vi "XP2i.vi"(4 "error in":T13, 7 "Command":T14) -> (0 "error out":T13, 3 "Response":T11)   [LabVIEW 2018]
uses:
  MOKO_LabViewLibrary/MokoLowLevel/MokoLowLovelControl/MLLC_Command.ctl
  MOKO_LabViewLibrary/MokoLowLevel/MokoLowLovelControl/MLLC_Error.ctl
  MOKO_LabViewLibrary/MokoLowLevel/MokoLowLovelControl/MLLC_Mode.ctl
  MOKO_LabViewLibrary/MokoLowLevel/MokoLowLovelControl/MLLC_Response.ctl
  MOKO_LabViewLibrary/MokoLowLevel/MokoLowLovelControl/MLLC_DriverName.ctl
  MOKO_LabViewLibrary/MokoLowLevel/MokoLowLovelControl/MLLC_ResponseInit.ctl
  MOKO_LabViewLibrary/MokoLowLevel/MokoLowLovelControl/MLLC_Request.ctl
  MOKO_LabViewLibrary/MokoLowLevel/MokoLowLovelControl/MLLC_ErrorCode.ctl
  MOKO_LabViewLibrary/MokoLowLevel/MokoLowLovelControl/MLLC_ConnectCluster.ctl
  MOKO_LabViewLibrary/MokoLowLevel/MokoLowLovelControl/MLLC_InterfaceType.ctl
  MOKO_LabViewLibrary/MokoLowLevel/MokoLowLovelControl/MLLC_OpenedSession.ctl
  MOKO_LabViewLibrary/MokoLowLevel/MokoLowLovelControl/MLLC_InterfaceSettings.ctl
  MOKO_LabViewLibrary/MokoLowLevel/MokoLowLovelControl/MLLC_InterfaceKind.ctl
  MOKO_LabViewLibrary/MokoLowLevel/MokoLowLovelControl/MLLC_Rs232Settings.ctl
panel:
  in  "Settings":T6={"Saved Data"=variant, "Permanent data"={"Connect"={"InterfaceType"=enum."VISA", "OpenedSession"="COM4", "InterfaceSettings"={"Interface"=enum."RS232", "EOS 4 read"=enum."Default (=EOS 4 write)", "EOS 4 write"=enum."CR (\\r)", "TMO, ms"=2000, "Sett"=variant(cluster{"Baud Rate":u32, "Data Bits":u16, "Parity":u16, "Stop Bits":u16, "Flow Control":u16, "Eho":bool} {"Baud Rate"=75, "Data Bits"=0, "Parity"=0, "Stop Bits"=0, "Flow Control"=0, "Eho"=FALSE})}}}}
  in  "Error Code":T7=5420
  in  "Request":T8="?MOD"
  in  "ResponseInit":T9="XP2I"
  in  "Driver Name":T10="Crystal XP2"
  in  "Mode":T12=enum."Check"
  # "XP2i"
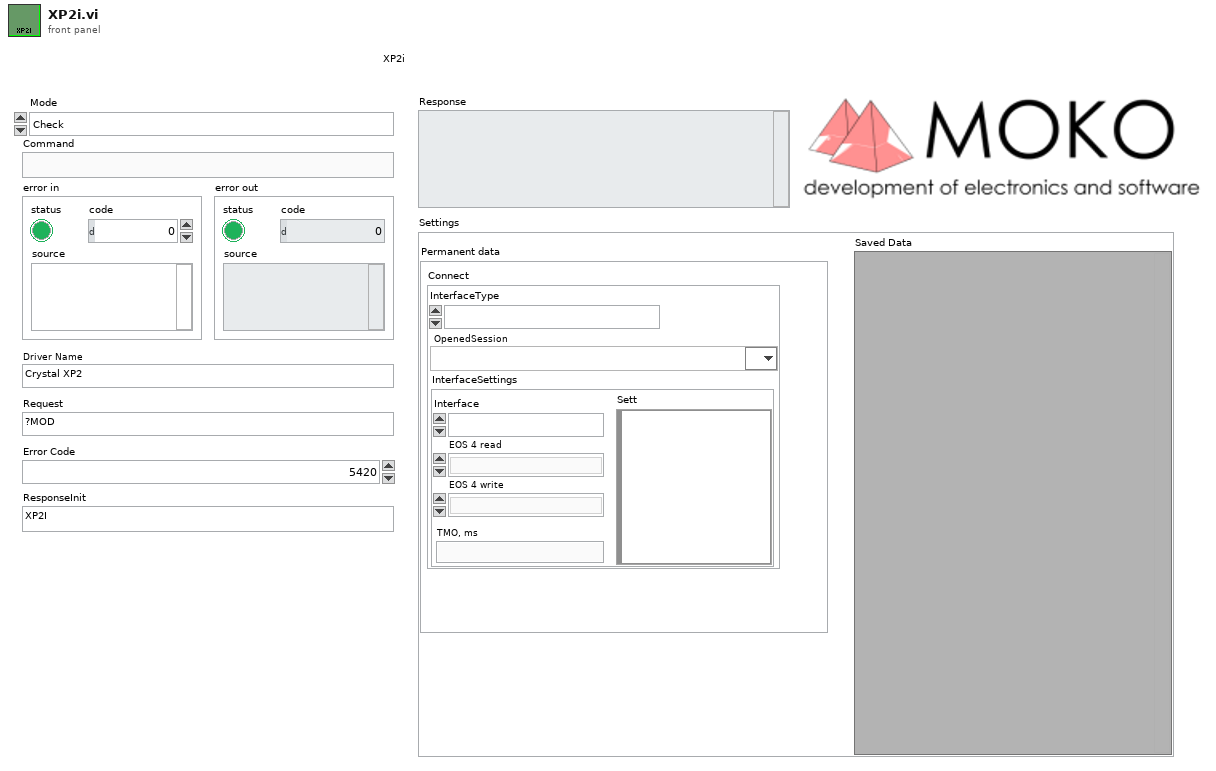
[diagram p1: front panel]
types:
  T1 = typedef "MLLC_ConnectCluster.ctl" = cluster{"InterfaceType":T2, "OpenedSession":T3, "InterfaceSettings":T4}
  T2 = typedef "MLLC_InterfaceType.ctl" = enum16{"VISA", "Prologix USB-GPIB"}
  T3 = typedef "MLLC_OpenedSession.ctl" = refnum<visa-resource-name>
  T4 = typedef "MLLC_InterfaceSettings.ctl" = cluster{"Interface":T5, "EOS 4 read":enum16{"Default (=EOS 4 write)", "CR (\\r)", "LF (\\n)", "None"}, "EOS 4 write":enum16{"CR+LF (\\r\\n)", "CR (\\r)", "LF (\\n)", "None"}, "TMO, ms":i32, "Sett":variant}
  T5 = typedef "MLLC_InterfaceKind.ctl" = enum16{"RS232", "GPIB", "USB", "Ethernet", "another"}
  T6 = cluster{"Saved Data":variant, "Permanent data":cluster{"Connect":T1}}
  T7 = typedef "MLLC_ErrorCode.ctl" = u32
  T8 = typedef "MLLC_Request.ctl" = string
  T9 = typedef "MLLC_ResponseInit.ctl" = string
  T10 = typedef "MLLC_DriverName.ctl" = string
  T11 = typedef "MLLC_Response.ctl" = string
  T12 = typedef "MLLC_Mode.ctl" = enum16{"get", "set", "close", "Init", "Check"}
  T13 = typedef "MLLC_Error.ctl" = errorcluster
  T14 = typedef "MLLC_Command.ctl" = string
  T15 = typedef "MLLC_Rs232Settings.ctl" = cluster{"Baud Rate":u32, "Data Bits":u16, "Parity":u16, "Stop Bits":u16, "Flow Control":u16, "Eho":bool}
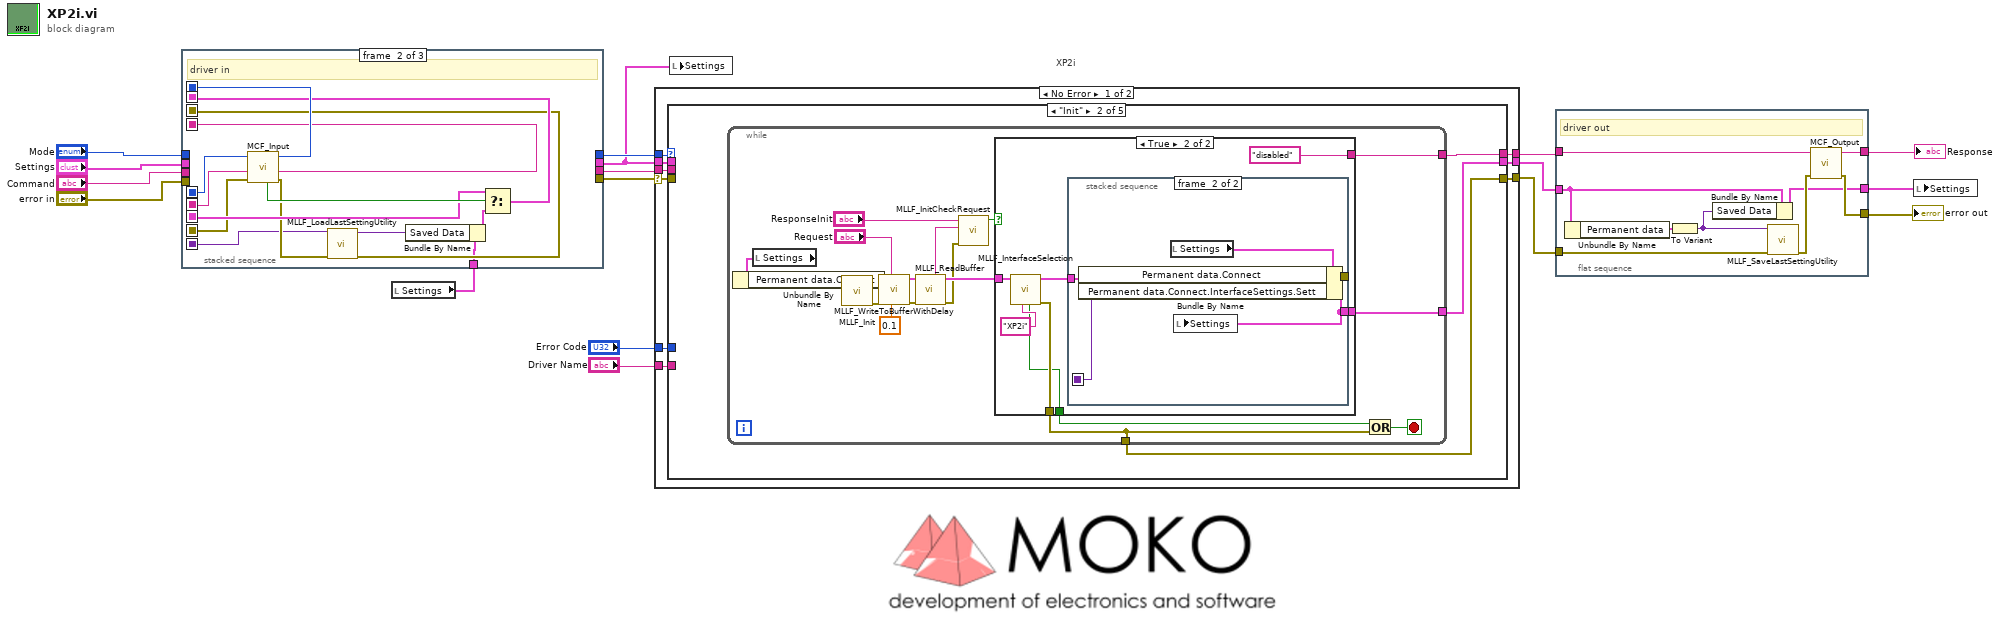
[diagram p0: block diagram]
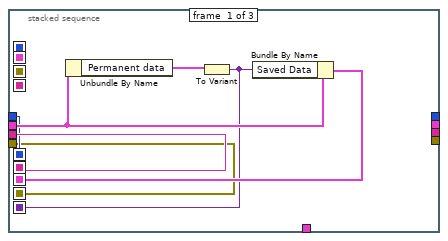
[diagram p2: hidden frame]
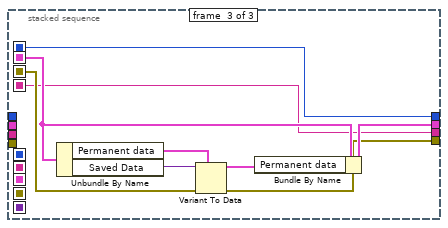
[diagram p3: hidden frame]
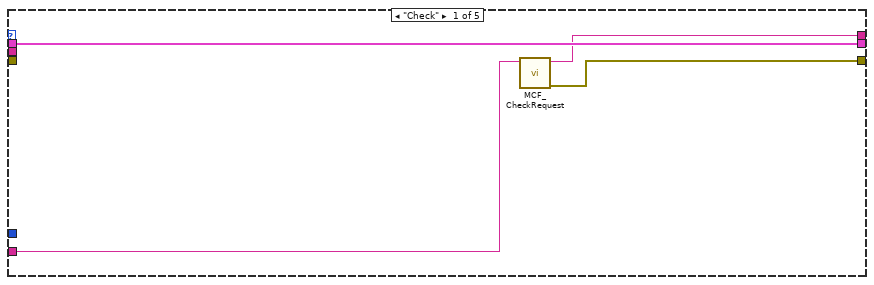
[diagram p4: hidden frame]
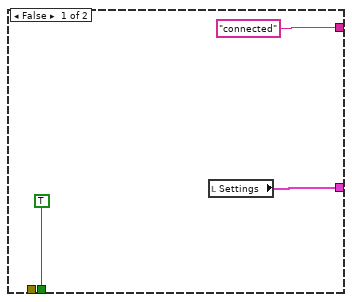
[diagram p5: hidden frame]
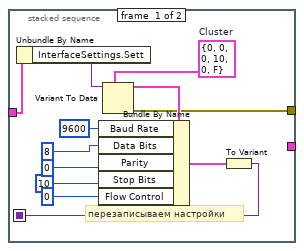
[diagram p6: hidden frame]
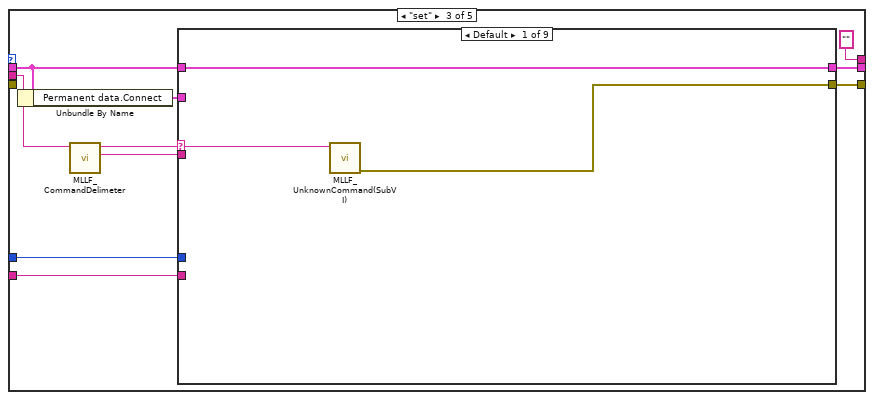
[diagram p7: hidden frame]
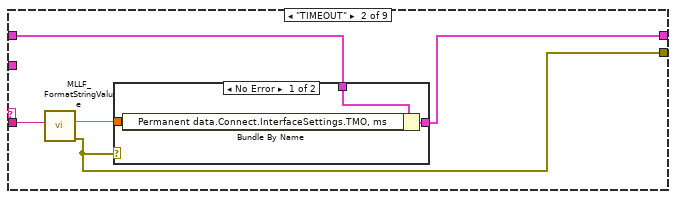
[diagram p8: hidden frame]
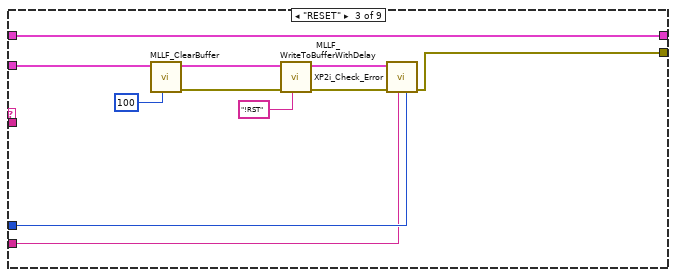
[diagram p10: hidden frame]
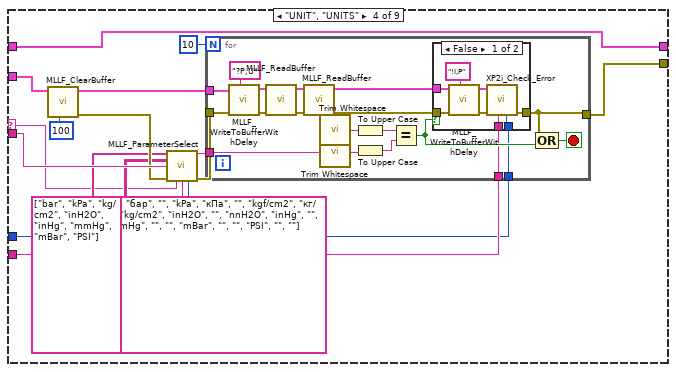
[diagram p11: hidden frame]
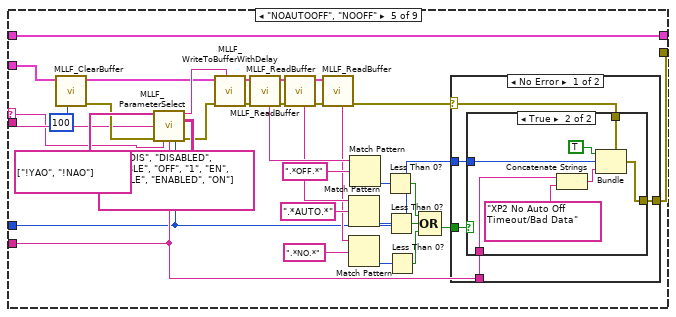
[diagram p13: hidden frame]
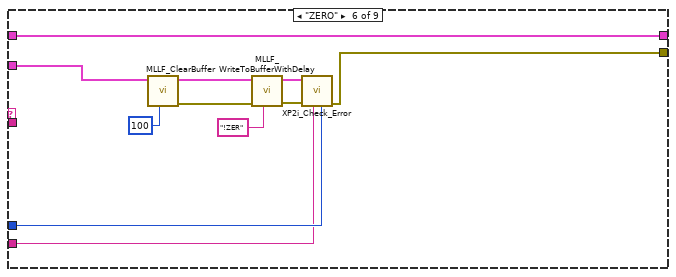
[diagram p16: hidden frame]
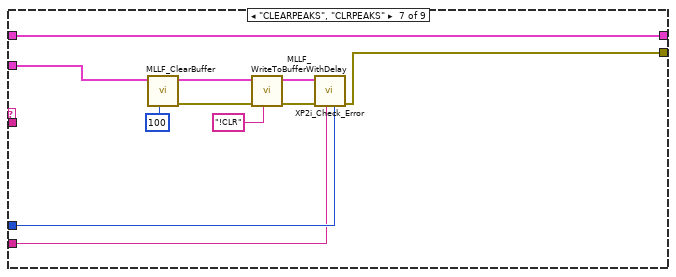
[diagram p17: hidden frame]
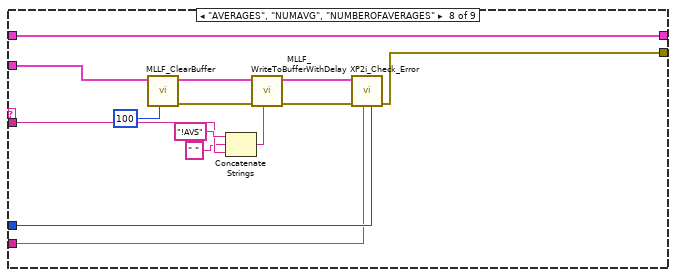
[diagram p18: hidden frame]
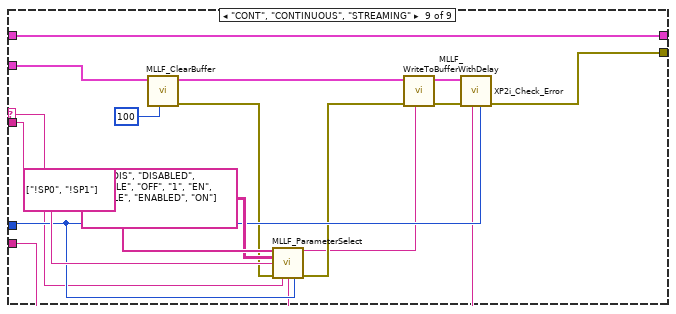
[diagram p19: hidden frame]
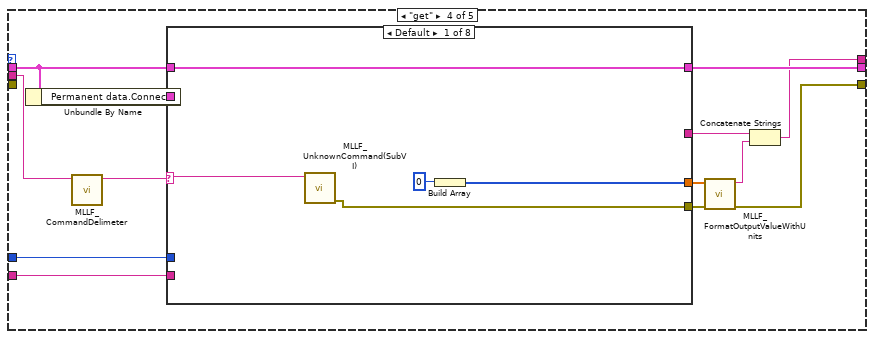
[diagram p20: hidden frame]
diagram:
  # "XP2i"
  n1 = local read "Settings"() -> (w7:T6)
  n2 = stacked-sequence {
    seq-local: [w20 _ _] -> [_ w36 _]
    seq-local: [w19 _ _] -> [_ w37 _]
    seq-local: [w22 _ _] -> [_ w32 _]
    seq-local: [w18 _ _] -> [_ w31 _]
    seq-local: [w21 _ _] -> [_ w27 _]
    seq-local: [_ w28 _] -> [_ _ w44]
    seq-local: [_ w38 _] -> [_ _ w41]
    seq-local: [_ w35 _] -> [_ _ w40]
    seq-local: [_ w34 _] -> [_ _ w45]
    tunnel: "Command" -> [w20 _ _]
    tunnel: "Mode" -> [w19 _ _]
    tunnel: "error in" -> [w18 _ _]
    tunnel: "Settings" -> [w23 _ _]
    tunnel: w7 -> [_ w26 _]
    tunnel: [_ _ w40] -> w9
    tunnel: [_ _ w43] -> w10
    tunnel: [_ _ w42] -> w8
    tunnel: [_ _ w41] -> w11
    frame #0 {
      n3 = Unbundle By Name(w23) -> ("Permanent data"=w24:cluster{"Connect":T1})
      n4 = To Variant(anything=w24) -> (Variant=w21:variant)
      n5 = Bundle By Name(cluster=w23, "Saved Data"=w21) -> (w22:T6)
    }
    frame #1 {
      # "driver in"
      n6 = call "MCF_Input.vi"("Error In"=w31, "Command in"=w36, "Mode in"=w37) -> ("Error Out"=w30:errorcluster, "Command out"=w35:string, "Mode out"=w38:T12, "Boolean"=w33:bool)  [unwired: 5 in]
      n7 = call "MLLF_LoadLastSettingUtility.vi"("Error In"=w30, "Save data in"=w27) -> ("Error Out"=w28:errorcluster, "Save data out"=w25:variant)  [unwired: 8 in]
      n8 = Bundle By Name(cluster=w26, "Saved Data"=w25) -> (w29:T6)
      n9 = Select(t=w32, s=w33, f=w29) -> (s? t:f=w34:T6)
    }
    frame #2 {
      n10 = Unbundle By Name(w45) -> ("Permanent data"=w46:cluster{"Connect":T1}, "Saved Data"=w39:variant)
      n11 = Variant To Data(error in=w44, type=w46, Variant=w39) -> (data=w47:cluster{"Connect":T1}, error out=w42:errorcluster)
      n12 = Bundle By Name(cluster=w45, "Permanent data"=w47) -> (w43:T6)
    }
  }
  n13 = case shown="No Error" w8 {
    selector: w8 -> [w53 w409]
    tunnel: [w48 w409] -> w4
    tunnel: w11 -> [w56 _]
    tunnel: [w55 _] -> w6
    tunnel: w9 -> [w54 _]
    tunnel: w10 -> [w50 w408]
    tunnel: "Error Code" -> [w52 _]
    tunnel: "Driver Name" -> [w51 _]
    tunnel: [w49 w408] -> w5
    frame No Error {
      n14 = case shown="\"Init\"" w56 {
        tunnel: [w58 w63 "" ("Output String") w293 "" ("Output String")] -> w55
        tunnel: w54 -> [_ _ w110 w286 _]
        tunnel: w53 -> [_ _ _ _ _]
        tunnel: w52 -> [_ _ w117 w296 _]
        tunnel: w51 -> [w59 _ w114 w295 _]
        tunnel: w50 -> [w60 _ w116 w297 w406]
        tunnel: [w60 w62 w115 w294 w406] -> w49
        tunnel: [w57 w61 w113 w287 w405] -> w48
        frame "Check" {
          n15 = call "MCF_CheckRequest.vi"("Driver Name"=w59) -> ("Error Out"=w57:errorcluster, "Output String"=w58:string)  [unwired: 9 in]
        }
        frame "Init" {
          n16 = while {
            tunnel: [w76] -> w61
            tunnel: [w73] -> w63
            tunnel: [w72] -> w62
            stop <- w78 stop-if-true
            n17 = local read "Settings"() -> (w66:T6)
            n18 = Unbundle By Name(w66) -> ("Permanent data.Connect"=w65:T1)
            n19 = call "MLLF_Init.vi"("DriverConnect in"=w65) -> ("Error Out"=w80:errorcluster, "DriverConnect out"=w79:T1)  [unwired: 7 in]
            n20 = call "MLLF_WriteToBufferWithDelay.vi"("Delay Time ( 0,05 s)"=0.1 ("Delay Time (s)"), "Command"="Request", "Error In"=w80, "DriverConnect in"=w79) -> ("Error Out"=w75:errorcluster, "DriverConnect out"=w64:T1)  [unwired: 6 in]
            n21 = call "MLLF_ReadBuffer.vi"("Error In"=w75, "DriverConnect in"=w64) -> ("Error Out"=w70:errorcluster, "DriverConnect out"=w81:T1, "String"=w71:string)  [unwired: 6 in]
            n22 = call "MLLF_InitCheckRequest.vi"("error in (no error)"=w70, "Answer"=w71, "Response Init"="ResponseInit") -> ("Design"=w69:bool)  [unwired: 5 in, 3 out]
            n23 = case shown="True" w69 {
              tunnel: w81 -> [_ w90]
              tunnel: [TRUE w86] -> w77
              tunnel: [_ w91] -> w76
              tunnel: ["connected" "disabled"] -> w73
              tunnel: [w82 w85] -> w72
              frame False {
                n24 = local read "Settings"() -> (w82:T6)
              }
              frame True {
                n25 = call "MLLF_InterfaceSelection.vi"("Driver Name"="XP2i" ("String"), "DriverConnect in"=w90) -> ("error out"=w91:T13, "DriverConnect out"=w89:T1, "stop init?"=w86:bool)  [unwired: 7 in]
                n26 = stacked-sequence {
                  seq-local: [w95 _] -> [_ w104]
                  tunnel: w89 -> [w93 w105]
                  tunnel: [w96 _] -> _
                  tunnel: [_ w106] -> w85
                  frame #0 {
                    w97 = T15 {"Baud Rate"=0, "Data Bits"=0, "Parity"=0, "Stop Bits"=10, "Flow Control"=0, "Eho"=FALSE}  # Cluster
                    # "перезаписываем настройки"
                    n27 = Unbundle By Name(w93) -> ("InterfaceSettings.Sett"=w92:variant)
                    n28 = Variant To Data(type=w97, Variant=w92) -> (data=w98:T15, error out=w96:errorcluster)  [unwired: 1 in]
                    n29 = Bundle By Name(cluster=w98, "Baud Rate"=u32 9600, "Data Bits"=u16 8 ("Serial Settings:Data Bits"), "Parity"=u16 0 ("Serial Settings:Parity"), "Stop Bits"=u16 10 ("Serial Settings:Stop Bits"), "Flow Control"=u16 0 ("Serial Settings:Flow Control")) -> (w103:T15)
                    n30 = To Variant(anything=w103) -> (Variant=w95:variant)
                  }
                  frame #1 {
                    n31 = local read "Settings"() -> (w107:T6)
                    n32 = Bundle By Name(cluster=w107, "Permanent data.Connect"=w105, "Permanent data.Connect.InterfaceSettings.Sett"=w104) -> (w106:T6)
                    n33 = local write "Settings"(w106) -> ()
                  }
                }
              }
            }
            n34 = Or(x=w77, y=w76) -> (x .or. y?=w78:bool)
          }
        }
        frame "set" {
          n35 = Unbundle By Name(w116) -> ("Permanent data.Connect"=w111:T1)
          n36 = call "MLLF_CommandDelimeter.vi"("command with param"=w110) -> ("param 1"=w108:string, "command"=w109:string)  [unwired: 6 in, 3 out]
          n37 = case shown="Default" w109 {
            selector: w109 -> [w119 _ _ w141 w185 _ _ _ w270]
            tunnel: w108 -> [_ w123 _ w153 w193 _ _ w260 w279]
            tunnel: w117 -> [_ _ w138 w151 w195 w238 w249 w264 w278]
            tunnel: w116 -> [w120 w124 w140 w144 w218 w243 w254 w268 w284]
            tunnel: [w120 w125 w140 w144 w218 w243 w254 w268 w284] -> w115
            tunnel: w114 -> [_ _ w137 w152 w196 w237 w248 w263 w269]
            tunnel: w111 -> [_ _ w131 w143 w187 w234 w245 w256 w272]
            tunnel: [w118 w121 w130 w142 w186 w233 w244 w255 w271] -> w113
            frame Default {
              n38 = call "MLLF_UnknownCommand(SubVI).vi"("Unknown command"=w119) -> ("error out"=w118:errorcluster)  [unwired: 10 in]
            }
            frame "TIMEOUT" {
              n39 = call "MLLF_FormatStringValue.vi"("String Value"=w123) -> ("error out"=w121:T13, "number"=w122:dbl)  [unwired: 8 in, 1 out]
              n40 = case shown="No Error" w121 {
                tunnel: [w128 w129] -> w125
                tunnel: w124 -> [w127 w129]
                tunnel: w122 -> [w126 _]
                frame No Error {
                  n41 = Bundle By Name(cluster=w127, "Permanent data.Connect.InterfaceSettings.TMO, ms"=w126) -> (w128:T6)
                }
                frame Error {
                }
              }
            }
            frame "RESET" {
              n42 = call "MLLF_ClearBuffer.vi"("Timeout"=u32 100, "DriverConnect in"=w131) -> ("Error Out"=w135:errorcluster, "DriverConnect out"=w134:T1)  [unwired: 6 in, 1 out]
              n43 = call "MLLF_WriteToBufferWithDelay.vi"("Command"="!RST" ("String"), "Error In"=w135, "DriverConnect in"=w134) -> ("Error Out"=w133:errorcluster, "DriverConnect out"=w139:T1)  [unwired: 7 in]
              n44 = call "XP2i_Check_Error.vi"("Error Code"=w138, "Driver Name"=w137, "Error In"=w133, "DriverConnect in"=w139) -> ("Error Out"=w130:errorcluster)  [unwired: 6 in, 1 out]
            }
            frame "UNIT", "UNITS" {
              n45 = call "MLLF_ClearBuffer.vi"("Timeout"=u32 100, "DriverConnect in"=w143) -> ("Error Out"=w150:errorcluster, "DriverConnect out"=w154:T1)  [unwired: 6 in, 1 out]
              n46 = call "MLLF_ParameterSelect.vi"("Command to equipment"=string[] ["bar", "kPa", "kg/cm2", "inH2O", "inHg", "mmHg", "mBar", "PSI"] ("Parameters 2 equipment"), "Names"=string[][] [["bar", "бар", ""], ["kPa", "кПа", ""], ["kgf/cm2", "кг/см2", "kg/cm2"], ["inH2O", "", "nnH2O"], ["inHg", "", ""], ["mmHg", "", ""], ["mBar", "", ""], ["PSI", "", ""]], "Input"=w153, "Error In"=w150, "Command"=w141, "Driver Name"=w152, "Error Code"=w151) -> ("Choice"=w148:string, "Error Out"=w149:errorcluster)  [unwired: 7 in]
              n47 = for {
                N: 10 -> [_]
                tunnel: w154 -> [w165]
                tunnel: [w159] -> w142
                tunnel: w148 -> [w163]
                tunnel: w152 -> [w157]
                tunnel: w151 -> [w156]
                tunnel: w149 -> [w164]
                stop <- w171 stop-if-true
                n48 = call "MLLF_WriteToBufferWithDelay.vi"("Command"="?P,U" ("String"), "Error In"=w164, "DriverConnect in"=w165) -> ("Error Out"=w167:errorcluster, "DriverConnect out"=w174:T1)  [unwired: 7 in]
                n49 = call "MLLF_ReadBuffer.vi"("Error In"=w167, "DriverConnect in"=w174) -> ("Error Out"=w170:errorcluster, "DriverConnect out"=w169:T1)  [unwired: 6 in, 1 out]
                n50 = call "MLLF_ReadBuffer.vi"("Error In"=w170, "DriverConnect in"=w169) -> ("Error Out"=w160:errorcluster, "DriverConnect out"=w161:T1, "String"=w168:string)  [unwired: 6 in]
                n51 = call <vilib>:"Trim Whitespace.vi"("string"=w168) -> ("trimmed string"=w166:string)  [unwired: 1 in]
                n52 = call <vilib>:"Trim Whitespace.vi"("string"=w163) -> ("trimmed string"=w162:string)  [unwired: 1 in]
                n53 = To Upper Case(1:w166) -> (0:w173:string)
                n54 = To Upper Case(1:w162) -> (0:w172:string)
                n55 = Equal?(x=w173, y=w172) -> (x = y?=w158:bool)
                n56 = case shown="False" w158 {
                  tunnel: w161 -> [w180 _]
                  tunnel: w160 -> [w179 w184]
                  tunnel: [w178 w184] -> w159
                  tunnel: w157 -> [w177 _]
                  tunnel: w156 -> [w176 _]
                  frame False {
                    n57 = call "MLLF_WriteToBufferWithDelay.vi"("Command"="!I,P" ("String"), "Error In"=w179, "DriverConnect in"=w180) -> ("Error Out"=w181:errorcluster, "DriverConnect out"=w182:T1)  [unwired: 7 in]
                    n58 = call "XP2i_Check_Error.vi"("Error Code"=w176, "Driver Name"=w177, "Error In"=w181, "DriverConnect in"=w182) -> ("Error Out"=w178:errorcluster)  [unwired: 6 in, 1 out]
                  }
                  frame True {
                  }
                }
                n59 = Compound Arithmetic op=OR(w159, w158) -> (w171:bool)
              }
            }
            frame "NOAUTOOFF", "NOOFF" {
              n60 = call "MLLF_ClearBuffer.vi"("Timeout"=u32 100, "DriverConnect in"=w187) -> ("Error Out"=w194:errorcluster, "DriverConnect out"=w190:T1)  [unwired: 6 in, 1 out]
              n61 = call "MLLF_ParameterSelect.vi"("Command to equipment"=string[] ["!YAO", "!NAO"] ("Names"), "Names"=string[][] [["0", "DIS", "DISABLED", "DISABLE", "OFF"], ["1", "EN", "ENABLE", "ENABLED", "ON"]], "Input"=w193, "Error In"=w194, "Command"=w185, "Driver Name"=w196, "Error Code"=w195) -> ("Choice"=w192:string, "Error Out"=w191:errorcluster)  [unwired: 7 in]
              n62 = call "MLLF_WriteToBufferWithDelay.vi"("Command"=w192, "Error In"=w191, "DriverConnect in"=w190) -> ("Error Out"=w188:errorcluster, "DriverConnect out"=w217:T1)  [unwired: 7 in]
              n63 = call "MLLF_ReadBuffer.vi"("Error In"=w188, "DriverConnect in"=w217) -> ("Error Out"=w216:errorcluster, "DriverConnect out"=w215:T1, "String"=w203:string)  [unwired: 6 in]
              n64 = call "MLLF_ReadBuffer.vi"("Error In"=w216, "DriverConnect in"=w215) -> ("Error Out"=w214:errorcluster, "DriverConnect out"=w213:T1, "String"=w202:string)  [unwired: 6 in]
              n65 = call "MLLF_ReadBuffer.vi"("Error In"=w214, "DriverConnect in"=w213) -> ("Error Out"=w200:errorcluster, "String"=w201:string)  [unwired: 6 in, 1 out]
              n66 = Match Pattern(string=w202, regular expression=".*AUTO.*") -> (offset past match=w208:i32)  [unwired: 1 in, 3 out]
              n67 = Match Pattern(string=w201, regular expression=".*NO.*") -> (offset past match=w209:i32)  [unwired: 1 in, 3 out]
              n68 = Match Pattern(string=w203, regular expression=".*OFF.*") -> (offset past match=w207:i32)  [unwired: 1 in, 3 out]
              n69 = Less Than 0?(x=w207) -> (x < 0?=w210:bool)
              n70 = Less Than 0?(x=w208) -> (x < 0?=w211:bool)
              n71 = Less Than 0?(x=w209) -> (x < 0?=w212:bool)
              n72 = Compound Arithmetic op=OR(w210, w211, w212) -> (w199:bool)
              n73 = case shown="No Error" w200 {
                selector: w200 -> [w219 w232]
                tunnel: [w223 w232] -> w186
                tunnel: w199 -> [w222 _]
                tunnel: w195 -> [w221 _]
                tunnel: w196 -> [w220 _]
                frame No Error {
                  n74 = case shown="True" w222 {
                    tunnel: [w224 w230] -> w223
                    tunnel: w221 -> [_ w229]
                    tunnel: w220 -> [_ w227]
                    tunnel: w219 -> [w224 w225]
                    frame False {
                    }
                    frame True {
                      n75 = Concatenate Strings(w227, "XP2 No Auto Off Timeout/Bad Data") -> (w226:string)
                      n76 = Bundle(cluster=w225, "status"=TRUE, "code"=w229, "source"=w226) -> (w230:errorcluster)
                    }
                  }
                }
                frame Error {
                }
              }
            }
            frame "ZERO" {
              n77 = call "MLLF_ClearBuffer.vi"("Timeout"=u32 100, "DriverConnect in"=w234) -> ("Error Out"=w241:errorcluster, "DriverConnect out"=w240:T1)  [unwired: 6 in, 1 out]
              n78 = call "MLLF_WriteToBufferWithDelay.vi"("Command"="!ZER" ("String"), "Error In"=w241, "DriverConnect in"=w240) -> ("Error Out"=w235:errorcluster, "DriverConnect out"=w239:T1)  [unwired: 7 in]
              n79 = call "XP2i_Check_Error.vi"("Error Code"=w238, "Driver Name"=w237, "Error In"=w235, "DriverConnect in"=w239) -> ("Error Out"=w233:errorcluster)  [unwired: 6 in, 1 out]
            }
            frame "CLEARPEAKS", "CLRPEAKS" {
              n80 = call "MLLF_ClearBuffer.vi"("Timeout"=u32 100, "DriverConnect in"=w245) -> ("Error Out"=w252:errorcluster, "DriverConnect out"=w251:T1)  [unwired: 6 in, 1 out]
              n81 = call "MLLF_WriteToBufferWithDelay.vi"("Command"="!CLR" ("String"), "Error In"=w252, "DriverConnect in"=w251) -> ("Error Out"=w247:errorcluster, "DriverConnect out"=w250:T1)  [unwired: 7 in]
              n82 = call "XP2i_Check_Error.vi"("Error Code"=w249, "Driver Name"=w248, "Error In"=w247, "DriverConnect in"=w250) -> ("Error Out"=w244:errorcluster)  [unwired: 6 in, 1 out]
            }
            frame "AVERAGES", "NUMAVG", "NUMBEROFAVERAGES" {
              n83 = call "MLLF_ClearBuffer.vi"("Timeout"=u32 100, "DriverConnect in"=w256) -> ("Error Out"=w267:errorcluster, "DriverConnect out"=w266:T1)  [unwired: 6 in, 1 out]
              n84 = Concatenate Strings("!AVS" ("String"), " " ("string"), w260) -> (w261:string)
              n85 = call "MLLF_WriteToBufferWithDelay.vi"("Command"=w261, "Error In"=w267, "DriverConnect in"=w266) -> ("Error Out"=w258:errorcluster, "DriverConnect out"=w265:T1)  [unwired: 7 in]
              n86 = call "XP2i_Check_Error.vi"("Error Code"=w264, "Driver Name"=w263, "Error In"=w258, "DriverConnect in"=w265) -> ("Error Out"=w255:errorcluster)  [unwired: 6 in, 1 out]
            }
            frame "CONT", "CONTINUOUS", "STREAMING" {
              n87 = call "MLLF_ClearBuffer.vi"("Timeout"=u32 100, "DriverConnect in"=w272) -> ("Error Out"=w277:errorcluster, "DriverConnect out"=w283:T1)  [unwired: 6 in, 1 out]
              n88 = call "MLLF_ParameterSelect.vi"("Command to equipment"=string[] ["!SP0", "!SP1"] ("Names"), "Names"=string[][] [["0", "DIS", "DISABLED", "DISABLE", "OFF"], ["1", "EN", "ENABLE", "ENABLED", "ON"]], "Input"=w279, "Error In"=w277, "Command"=w270, "Driver Name"=w269, "Error Code"=w278) -> ("Choice"=w275:string, "Error Out"=w276:errorcluster)  [unwired: 7 in]
              n89 = call "MLLF_WriteToBufferWithDelay.vi"("Command"=w275, "Error In"=w276, "DriverConnect in"=w283) -> ("Error Out"=w274:errorcluster, "DriverConnect out"=w282:T1)  [unwired: 7 in]
              n90 = call "XP2i_Check_Error.vi"("Error Code"=w278, "Driver Name"=w269, "Error In"=w274, "DriverConnect in"=w282) -> ("Error Out"=w271:errorcluster)  [unwired: 6 in, 1 out]
            }
          }
        }
        frame "get" {
          n91 = Unbundle By Name(w297) -> ("Permanent data.Connect"=w288:T1)
          n92 = call "MLLF_CommandDelimeter.vi"("command with param"=w286) -> ("command"=w285:string)  [unwired: 6 in, 4 out]
          n93 = case shown="Default" w285 {
            selector: w285 -> [w299 _ _ _ _ _ _ _]
            tunnel: [w298 _ w314 w328 w345 w362 w379 w396] -> w292
            tunnel: w296 -> [_ _ _ _ _ _ _ _]
            tunnel: [w302 w305 w318 w335 w352 w369 w386 w403] -> w294
            tunnel: w297 -> [w302 w305 w318 w335 w352 w369 w386 w403]
            tunnel: [w300 w303 _ w332 w349 w366 w383 w400] -> w291
            tunnel: w295 -> [_ _ _ _ _ _ _ _]
            tunnel: [_ _ w309 _ _ _ _ _] -> w289
            tunnel: w288 -> [_ _ w306 w319 w336 w353 w370 w387]
            frame Default {
              n94 = call "MLLF_UnknownCommand(SubVI).vi"("Unknown command"=w299) -> ("error out"=w298:errorcluster)  [unwired: 10 in]
              n95 = Build Array(0 ("TimeOut")) -> (w300:i32[])
            }
            frame "TIMEOUT" {
              n96 = Unbundle By Name(w305) -> ("Permanent data.Connect.InterfaceSettings.TMO, ms"=w304:i32)
              n97 = Build Array(w304) -> (w303:i32[])
            }
            frame "PRESSURE" {
              n98 = call "MLLF_ClearBuffer.vi"("Timeout"=u32 100, "DriverConnect in"=w306) -> ("Error Out"=w315:errorcluster, "DriverConnect out"=w316:T1)  [unwired: 6 in, 1 out]
              n99 = call "MLLF_WriteToBufferWithDelay.vi"("Command"="?PRE" ("String"), "Error In"=w315, "DriverConnect in"=w316) -> ("Error Out"=w308:errorcluster, "DriverConnect out"=w313:T1)  [unwired: 7 in]
              n100 = call "MLLF_ReadBuffer.vi"("Error In"=w308, "DriverConnect in"=w313) -> ("Error Out"=w314:errorcluster, "String"=w312:string)  [unwired: 6 in, 1 out]
              n101 = Match Pattern(string=w312, regular expression=",") -> (before substring=w310:string)  [unwired: 1 in, 3 out]
              n102 = call <vilib>:"Trim Whitespace.vi"("string"=w310) -> ("trimmed string"=w309:string)  [unwired: 1 in]
            }
            frame "PRESSUREHIGH" {
              n103 = call "MLLF_ClearBuffer.vi"("Timeout"=u32 100, "DriverConnect in"=w319) -> ("Error Out"=w329:errorcluster, "DriverConnect out"=w330:T1)  [unwired: 6 in, 1 out]
              n104 = call "MLLF_WriteToBufferWithDelay.vi"("Command"="?P,H" ("String"), "Error In"=w329, "DriverConnect in"=w330) -> ("Error Out"=w321:errorcluster, "DriverConnect out"=w325:T1)  [unwired: 7 in]
              n105 = call "MLLF_ReadBuffer.vi"("Error In"=w321, "DriverConnect in"=w325) -> ("Error Out"=w324:errorcluster, "DriverConnect out"=w323:T1, "String"=w322:string)  [unwired: 6 in]
              n106 = call "MLLF_ReadBuffer.vi"("Error In"=w324, "DriverConnect in"=w323) -> ("Error Out"=w328:errorcluster)  [unwired: 6 in, 2 out]
              n107 = Match Pattern(string=w322, regular expression=",") -> (before substring=w326:string)  [unwired: 1 in, 3 out]
              n108 = Fract/Exp String To Number(use system decimal point (T)=FALSE, string=w326) -> (number=w333:dbl)  [unwired: 2 in, 1 out]
              n109 = Build Array(w333) -> (w332:dbl[])
            }
            frame "PRESSURELOW" {
              n110 = call "MLLF_ClearBuffer.vi"("Timeout"=u32 100, "DriverConnect in"=w336) -> ("Error Out"=w346:errorcluster, "DriverConnect out"=w347:T1)  [unwired: 6 in, 1 out]
              n111 = call "MLLF_WriteToBufferWithDelay.vi"("Command"="?P,L" ("String"), "Error In"=w346, "DriverConnect in"=w347) -> ("Error Out"=w338:errorcluster, "DriverConnect out"=w342:T1)  [unwired: 7 in]
              n112 = call "MLLF_ReadBuffer.vi"("Error In"=w338, "DriverConnect in"=w342) -> ("Error Out"=w341:errorcluster, "DriverConnect out"=w340:T1, "String"=w339:string)  [unwired: 6 in]
              n113 = call "MLLF_ReadBuffer.vi"("Error In"=w341, "DriverConnect in"=w340) -> ("Error Out"=w345:errorcluster)  [unwired: 6 in, 2 out]
              n114 = Match Pattern(string=w339, regular expression=",") -> (before substring=w343:string)  [unwired: 1 in, 3 out]
              n115 = Fract/Exp String To Number(use system decimal point (T)=FALSE, string=w343) -> (number=w350:dbl)  [unwired: 2 in, 1 out]
              n116 = Build Array(w350) -> (w349:dbl[])
            }
            frame "AVERAGEPRESSURE", "AVGPRESS", "AVGPRESSURE" {
              n117 = call "MLLF_ClearBuffer.vi"("Timeout"=u32 100, "DriverConnect in"=w353) -> ("Error Out"=w363:errorcluster, "DriverConnect out"=w364:T1)  [unwired: 6 in, 1 out]
              n118 = call "MLLF_WriteToBufferWithDelay.vi"("Command"="?P,A" ("String"), "Error In"=w363, "DriverConnect in"=w364) -> ("Error Out"=w355:errorcluster, "DriverConnect out"=w359:T1)  [unwired: 7 in]
              n119 = call "MLLF_ReadBuffer.vi"("Error In"=w355, "DriverConnect in"=w359) -> ("Error Out"=w358:errorcluster, "DriverConnect out"=w357:T1, "String"=w356:string)  [unwired: 6 in]
              n120 = call "MLLF_ReadBuffer.vi"("Error In"=w358, "DriverConnect in"=w357) -> ("Error Out"=w362:errorcluster)  [unwired: 6 in, 2 out]
              n121 = Match Pattern(string=w356, regular expression=",") -> (before substring=w360:string)  [unwired: 1 in, 3 out]
              n122 = Fract/Exp String To Number(use system decimal point (T)=FALSE, string=w360) -> (number=w367:dbl)  [unwired: 2 in, 1 out]
              n123 = Build Array(w367) -> (w366:dbl[])
            }
            frame "RANGE" {
              n124 = call "MLLF_ClearBuffer.vi"("Timeout"=u32 100, "DriverConnect in"=w370) -> ("Error Out"=w380:errorcluster, "DriverConnect out"=w381:T1)  [unwired: 6 in, 1 out]
              n125 = call "MLLF_WriteToBufferWithDelay.vi"("Command"="?RNG" ("String"), "Error In"=w380, "DriverConnect in"=w381) -> ("Error Out"=w372:errorcluster, "DriverConnect out"=w376:T1)  [unwired: 7 in]
              n126 = call "MLLF_ReadBuffer.vi"("Error In"=w372, "DriverConnect in"=w376) -> ("Error Out"=w375:errorcluster, "DriverConnect out"=w374:T1, "String"=w373:string)  [unwired: 6 in]
              n127 = call "MLLF_ReadBuffer.vi"("Error In"=w375, "DriverConnect in"=w374) -> ("Error Out"=w379:errorcluster)  [unwired: 6 in, 2 out]
              n128 = Match Pattern(string=w373, regular expression=",") -> (before substring=w377:string)  [unwired: 1 in, 3 out]
              n129 = Fract/Exp String To Number(use system decimal point (T)=FALSE, string=w377) -> (number=w384:dbl)  [unwired: 2 in, 1 out]
              n130 = Build Array(w384) -> (w383:dbl[])
            }
            frame "ZERO" {
              n131 = call "MLLF_ClearBuffer.vi"("Timeout"=u32 100, "DriverConnect in"=w387) -> ("Error Out"=w397:errorcluster, "DriverConnect out"=w398:T1)  [unwired: 6 in, 1 out]
              n132 = call "MLLF_WriteToBufferWithDelay.vi"("Command"="?Z,U" ("String"), "Error In"=w397, "DriverConnect in"=w398) -> ("Error Out"=w389:errorcluster, "DriverConnect out"=w393:T1)  [unwired: 7 in]
              n133 = call "MLLF_ReadBuffer.vi"("Error In"=w389, "DriverConnect in"=w393) -> ("Error Out"=w392:errorcluster, "DriverConnect out"=w391:T1, "String"=w390:string)  [unwired: 6 in]
              n134 = call "MLLF_ReadBuffer.vi"("Error In"=w392, "DriverConnect in"=w391) -> ("Error Out"=w396:errorcluster)  [unwired: 6 in, 2 out]
              n135 = Match Pattern(string=w390, regular expression=",") -> (before substring=w394:string)  [unwired: 1 in, 3 out]
              n136 = Fract/Exp String To Number(use system decimal point (T)=FALSE, string=w394) -> (number=w401:dbl)  [unwired: 2 in, 1 out]
              n137 = Build Array(w401) -> (w400:dbl[])
            }
          }
          n138 = call "MLLF_FormatOutputValueWithUnits.vi"("error in"=w292, "ValuesIn"=w291) -> ("error out"=w287:T13, "Result string"=w290:T14)  [unwired: 8 in]
          n139 = Concatenate Strings(w289, w290) -> (w293:string)
        }
        frame "close" {
          n140 = Unbundle By Name(w406) -> ("Permanent data.Connect.OpenedSession"=w407:T3)
          n141 = VISA Close(VISA resource name=w407) -> (error out=w405:errorcluster)  [unwired: 1 in]
        }
      }
    }
    frame Error {
    }
  }
  n142 = local write "Settings"(w10) -> ()
  n143 = flat-sequence {
    tunnel: [w418] -> w3
    tunnel: [w417] -> w1
    tunnel: w6 -> [w416]
    tunnel: w4 -> [w415]
    tunnel: w5 -> [w411]
    tunnel: [w413] -> w2
    frame #0 {
      # "driver out"
      n144 = Unbundle By Name(w411) -> ("Permanent data"=w410:cluster{"Connect":T1})
      n145 = To Variant(anything=w410) -> (Variant=w412:variant)
      n146 = Bundle By Name(cluster=w411, "Saved Data"=w412) -> (w413:T6)
      n147 = call "MLLF_SaveLastSettingUtility.vi"("error in"=w415, "Saved Data"=w412) -> ("error out"=w414:T13)  [unwired: 8 in, 1 out]
      n148 = call "MCF_Output.vi"("Error In"=w414, "Input"=w416) -> ("Error Out"=w417:errorcluster, "Output"=w418:string)  [unwired: 8 in]
    }
  }
  n149 = local write "Settings"(w2) -> ()
  "error out" <- w1
  "Response" <- w3
